vi "檔案.vi"() -> ()   [LabVIEW 2015]
panel:
  in  "Save As Button":bool
  in  "New Recipe":string
  in  "Delete Button":bool
  in  "Save Button":bool
  in  "Recipe Ring":u8(ring)
  in  "Exit":bool
  # "Recipe"
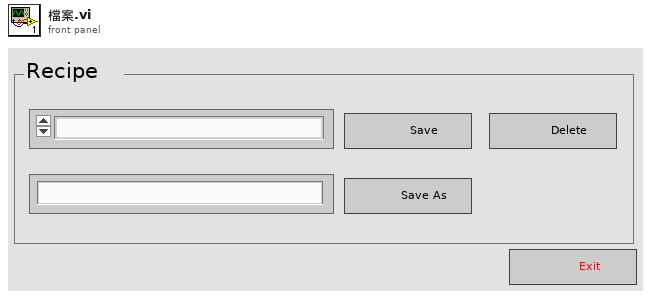
[diagram p1: front panel]
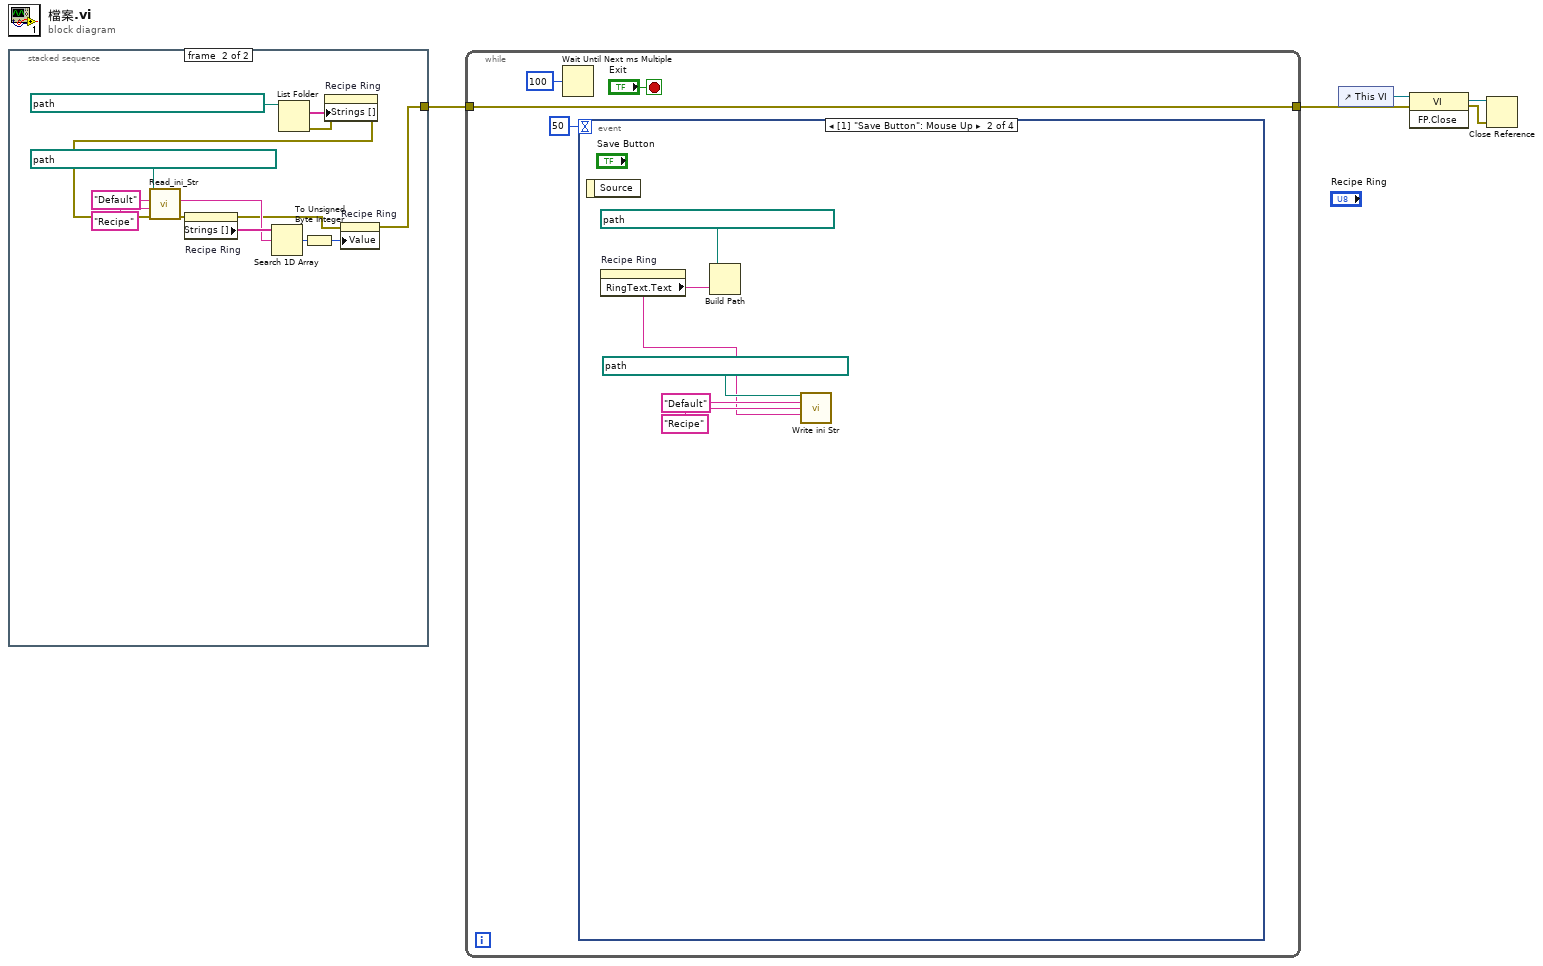
[diagram p0: block diagram]
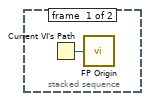
[diagram p2: hidden frame]
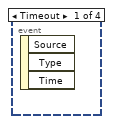
[diagram p3: hidden frame]
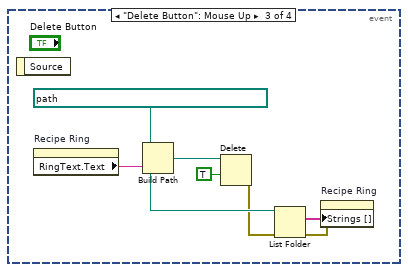
[diagram p4: hidden frame]
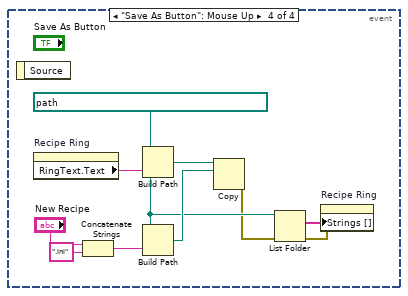
[diagram p5: hidden frame]
diagram:
  n1 = stacked-sequence {
    tunnel: [_ w7] -> w1
    frame #0 {
      n2 = Current VI's Path() -> (path=w6:path)
      n3 = call "FP Origin.vi"("vi path"=w6) -> ()  [unwired: 1 out]
    }
    frame #1 {
      n4 = List Folder(path=path "D:/Folding自動機 Data/Recipe/Position" ("configuration file path")) -> (filenames=w17:string[], error out=w15:errorcluster)  [unwired: 3 in, 2 out]
      n5 = property on="Recipe Ring" class="Ring (strict)"(error in=w15, "Strings []"=w17) -> (error out=w14:errorcluster)  [unwired: 1 in, 1 out]
      n6 = call "Read_ini_Str.vi"("error in (no error)"=w14, "key"="Recipe", "section"="Default", "configuration file path"=path "D:/Folding自動機 Data/Recipe/Default.ini") -> ("error out"=w13:errorcluster, "value"=w11:string)  [unwired: 6 in]
      n7 = property on="Recipe Ring" class="Ring (strict)"(error in=w13) -> (error out=w8:errorcluster, "Strings []"=w12:string[])  [unwired: 1 in, 1 out]
      n8 = Search 1D Array(1D array=w12, element=w11) -> (index of element=w10:i32)  [unwired: 1 in]
      n9 = To Unsigned Byte Integer(number=w10) -> (unsigned 8bit integer=w9:u8)
      n10 = property on="Recipe Ring" class="Ring (strict)"(error in=w8, "Value"=w9) -> (error out=w7:errorcluster)  [unwired: 1 in, 1 out]
    }
  }
  n11 = while {
    tunnel: w1 -> [w21]
    tunnel: [w21] -> w5
    stop <- "Exit" stop-if-true
    n12 = Wait Until Next ms Multiple(millisecond multiple=u32 100) -> ()  [unwired: 1 out]
    n13 = event shown="[1] \"Save Button\": Mouse Up" {
      selector: _ -> [_ _ _ _]
      dyn-events: _ -> [_ _ _ _]
      timeout: 50 -> [_ _ _ _]
      event Timeout {
        n14 = event-data() -> ()  [unwired: 1 in, 3 out]
      }
      event "Save Button": Mouse Up {
        n15 = event-data() -> ()  [unwired: 1 in, 1 out]
        n16 = property on="Recipe Ring" class="Ring (strict)"() -> ("RingText.Text"=w25:string)  [unwired: 2 in, 2 out]
        n17 = Build Path(base path=path "D:/Folding自動機 Data/Recipe/Position" ("configuration file path"), name or relative path=w25) -> ()  [unwired: 1 out]
        n18 = call "Write ini Str.vi"("configuration file path"=path "D:/Folding自動機 Data/Recipe/Default.ini", "section"="Default", "key"="Recipe", "value"=w25) -> ()  [unwired: 11 in, 1 out]
      }
      event "Delete Button": Mouse Up {
        w32 = path "D:/Folding自動機 Data/Recipe/Position" ("configuration file path")
        n19 = event-data() -> ()  [unwired: 1 in, 1 out]
        n20 = property on="Recipe Ring" class="Ring (strict)"() -> ("RingText.Text"=w36:string)  [unwired: 2 in, 2 out]
        n21 = Build Path(base path=w32, name or relative path=w36) -> (appended path=w35:path)
        n22 = Delete(path (use dialog)=w35, confirm (F)=TRUE) -> (error out=w31:errorcluster)  [unwired: 3 in, 2 out]
        n23 = List Folder(path=w32, error in=w31) -> (filenames=w33:string[], error out=w30:errorcluster)  [unwired: 2 in, 2 out]
        n24 = property on="Recipe Ring" class="Ring (strict)"(error in=w30, "Strings []"=w33) -> ()  [unwired: 1 in, 2 out]
      }
      event "Save As Button": Mouse Up {
        w38 = path "D:/Folding自動機 Data/Recipe/Position" ("configuration file path")
        n25 = event-data() -> ()  [unwired: 1 in, 1 out]
        n26 = property on="Recipe Ring" class="Ring (strict)"() -> ("RingText.Text"=w46:string)  [unwired: 2 in, 2 out]
        n27 = Concatenate Strings("New Recipe", ".ini" ("string")) -> (w40:string)
        n28 = Build Path(base path=w38, name or relative path=w46) -> (appended path=w43:path)
        n29 = Build Path(base path=w38, name or relative path=w40) -> (appended path=w39:path)
        n30 = Copy(10:w39, 11:w43) -> (0:w37:errorcluster)  [unwired: 3 in, 2 out]
        n31 = List Folder(path=w38, error in=w37) -> (filenames=w45:string[], error out=w44:errorcluster)  [unwired: 2 in, 2 out]
        n32 = property on="Recipe Ring" class="Ring (strict)"(error in=w44, "Strings []"=w45) -> ()  [unwired: 1 in, 2 out]
      }
    }
  }
  n33 = control-ref of="This VI"() -> (w4:refnum<vi>)
  n34 = invoke class="VI" method="FP.Close"(reference=w4, error in=w5) -> (reference out=w3:refnum<vi>, error out=w2:errorcluster)  [unwired: 1 in, 1 out]
  n35 = Close Reference(reference=w3, error in (no error)=w2) -> ()  [unwired: 1 out]
